vi "Read Decimated Traces.vi"(8 "Error In":errorcluster, 11 "BNT_DSCXYGraph in":refnum<class "BNT_DSCXYGraph.lvclass">) -> (0 "Error Out":errorcluster, 3 "BNT_DSCXYGraph out":refnum<class "BNT_DSCXYGraph.lvclass">)   [LabVIEW 2015, in "BNT_DSCXYGraph.lvlib" / "BNT_DSCXYGraph.lvclass"]
doc: "Read X-Y traces from DSC database."
uses:
  BNT_DSCXYGraph.lvclass
  BNT_DSCXYGraph.lvclass/BNT_DSCXYGraph.ctl
  <vilib>/lvdsc/historical/Read Traces (Numeric).vi
  <vilib>/lvdsc/NI_DSC.lvlib
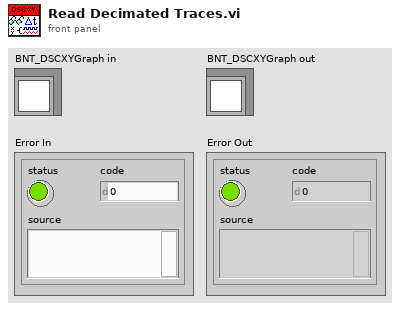
[diagram p1: front panel]
types:
  T1 = cluster{"interpolate data (F)":bool, "extrapolate to now (F)":bool, "remove data breaks (F)":bool, "interpolation interval (1 s)":dbl, "maintain trending info (T)":bool}
  T2 = cluster{"Start Time":timestamp, "seconds since 1Jan1904":timestamp}
  T3 = cluster{"timestamps":timestamp[], "data":dbl[]}[]
  T4 = cluster{"decimated traces":dbl[], "decimated traces":dbl[]}
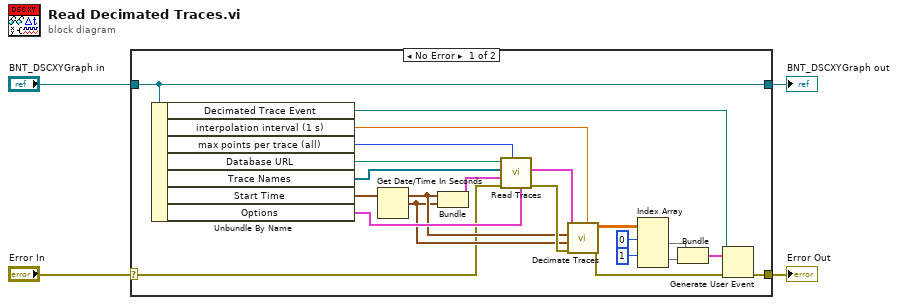
[diagram p0: block diagram]
diagram:
  n1 = case shown="No Error" "Error In" {
    selector: "Error In" -> [w10 w27]
    tunnel: [w6 w27] -> w3
    tunnel: [w25 w26] -> w1
    tunnel: "BNT_DSCXYGraph in" -> [w25 w26]
    frame No Error {
      n2 = Unbundle By Name(w25) -> ("Decimated Trace Event"=w8:refnum<user-event>, "interpolation interval (1 s)"=w15:dbl, "max points per trace (all)"=w20:i32, "Database URL"=w24:path, "Trace Names"=w23:refnum<k21>[], "Start Time"=w17:timestamp, "Options"=w21:T1)
      n3 = Get Date/Time In Seconds() -> (seconds since 1Jan1904=w16:timestamp)
      n4 = Bundle("Start Time"=w17, "seconds since 1Jan1904"=w16) -> (w22:T2)  [unwired: 1 in]
      n5 = call-poly <vilib>:"Read Traces.vi"("options"=w21, "max points per trace (all)"=w20, "error in (no error)"=w10, "time interval"=w22, "trace names"=w23, "database URL"=w24) -> ("error out"=w18:errorcluster, "historical traces"=w19:T3)  [unwired: 2 in, 2 out]
      n6 = call <vilib>:"Decimate Traces.vi"("sample interval"=w15, "error in (no error)"=w18, "stop timestamp"=w16, "start timestamp"=w17, "historical traces"=w19) -> ("error out"=w7:errorcluster, "decimated traces"=w9:dbl[][])  [unwired: 3 in, 2 out]
      n7 = Index Array(array=w9, index (row) #1=0 ("index (row)"), index (row) #2=1 ("index (row)")) -> (element #1=w13:dbl[], element #2=w14:dbl[])  [unwired: 2 in]
      n8 = Bundle("decimated traces"=w13, "decimated traces"=w14) -> (w5:T4)  [unwired: 1 in]
      n9 = Generate User Event(user event=w8, event data cluster=w5, error in=w7) -> (error out=w6:errorcluster)  [unwired: 1 in, 1 out]
    }
    frame Error {
    }
  }
  "Error Out" <- w3
  "BNT_DSCXYGraph out" <- w1
